vi "SET.vi"(0 "TCP session out":refnum<k5>, 1 "Key":string, 2 "Option":enum16{"None", "NX", "XX"}(ring), 5 "Value":string, 7 "Use EX ?":bool, 9 "Seconds":string, 11 "error in":errorcluster, 12 "Use PX ?":bool, 13 "Milliseconds":string) -> (4 "TCP session out":refnum<k5>, 6 "Data":T1, 15 "error out":errorcluster)   [LabVIEW 2023]
uses:
  SubVIs/Controls/redis-data.ctl
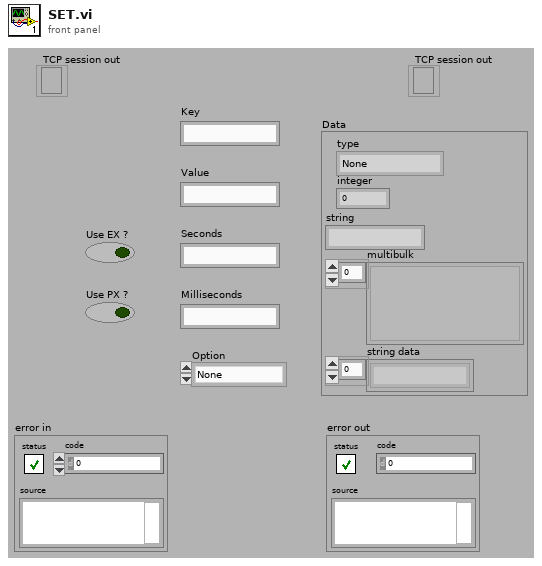
[diagram p1: front panel]
types:
  T1 = typedef "redis-data.ctl" = cluster{"type":enum16{"None", "Error", "Status", "Nil", "Integer", "String", "Multibulk"}, "integer":i64, "string":string, "multibulk":variant[], "string data":string[]}
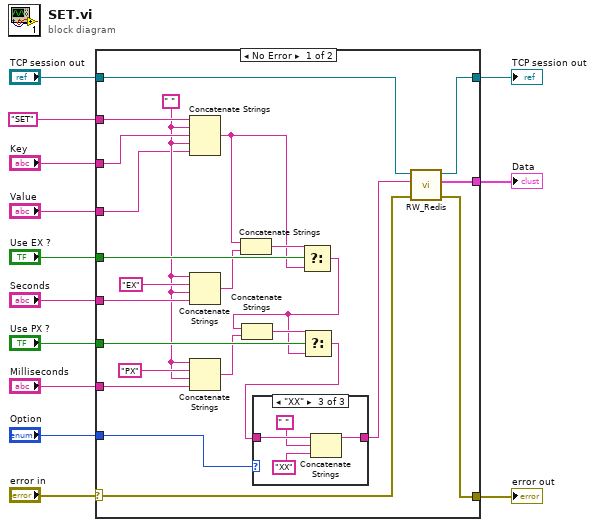
[diagram p0: block diagram]
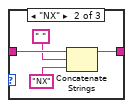
[diagram p3: hidden frame]
diagram:
  n1 = case shown="No Error" "error in" {
    selector: "error in" -> [w36 w48]
    tunnel: "Key" -> [w33 _]
    tunnel: "SET" -> [w37 _]
    tunnel: "TCP session out" -> [w20 w47]
    tunnel: [w35 w48] -> w11
    tunnel: [w34 _] -> w3
    tunnel: "Seconds" -> [w32 _]
    tunnel: "Use EX ?" -> [w30 _]
    tunnel: "Use PX ?" -> [w23 _]
    tunnel: "Milliseconds" -> [w28 _]
    tunnel: [w14 w47] -> w5
    tunnel: "Value" -> [w18 _]
    tunnel: "Option" -> [w17 _]
    frame No Error {
      w19 = " "
      n2 = Concatenate Strings(w37, w19, w33, w19, w18) -> (w26:string)
      n3 = Concatenate Strings(w19, "EX", w19, w32) -> (w25:string)
      n4 = Concatenate Strings(w19, "PX", w19, w28) -> (w21:string)
      n5 = Concatenate Strings(w26, w25) -> (w27:string)
      n6 = Select(t=w27, s=w30, f=w26) -> (s? t:f=w22:string)
      n7 = Concatenate Strings(w22, w21) -> (w24:string)
      n8 = Select(t=w24, s=w23, f=w22) -> (s? t:f=w16:string)
      n9 = case shown="\"XX\"" w17 {
        tunnel: w16 -> [w38 w42 w46]
        tunnel: [w38 w39 w43] -> w15
        frame "None", Default {
        }
        frame "NX" {
          n10 = Concatenate Strings(w42, " ", "NX") -> (w39:string)
        }
        frame "XX" {
          n11 = Concatenate Strings(w46, " ", "XX") -> (w43:string)
        }
      }
      n12 = call "RW_Redis.vi"("error in"=w36, "command"=w15, "TCP session in"=w20) -> ("error out"=w35:errorcluster, "Data"=w34:T1, "TCP session out"=w14:refnum<k5>)  [unwired: 6 in]
    }
    frame Error {
    }
  }
  "error out" <- w11
  "Data" <- w3
  "TCP session out" <- w5
